vi "Ball Ball Velocity after Collision Calcul.vi"(10 "Movables in":refnum<class "Movable.lvclass">[](array[class])) -> (2 "Movables out":refnum<class "Movable.lvclass">[](array[class]))   [LabVIEW 2024, in "Game Board.lvclass"]
doc: "MIT Licence\nCopyright (c) 2024 David Grollier"
uses:
  Game Board.lvclass
  Game Board Component/Movable/Movable.lvclass
  Game Board Component/Movable/Movable.lvclass/Movable.ctl
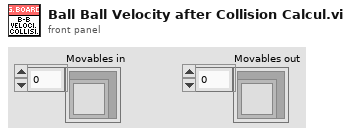
[diagram p1: front panel]
types:
  T1 = typedef "Coordinates.ctl" = cluster{"x":dbl, "y":dbl}
  T2 = typedef "Velocity.ctl" = cluster{"Vx":dbl, "Vy":dbl}
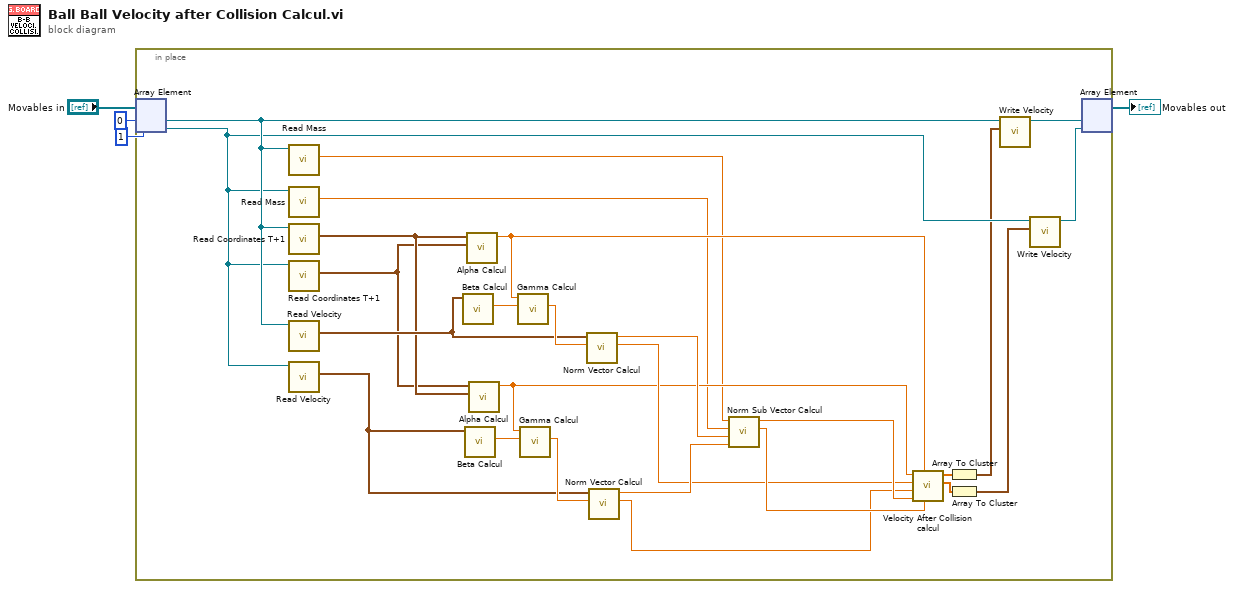
[diagram p0: block diagram]
diagram:
  n1 = in-place {
    n2 = in-place-array #1("Movables in", 0, 1) -> (w12:refnum<class "Movable.lvclass">, w11:refnum<class "Movable.lvclass">)
    n3 = call "Read Mass.vi"("Movable in"=w12) -> ("Mass"=w16:dbl)  [unwired: 10 in]
    n4 = call "Read Mass.vi"("Movable in"=w11) -> ("Mass"=w15:dbl)  [unwired: 10 in]
    n5 = call "Read Coordinates T+1.vi"("Movable in"=w12) -> ("Coordinates"=w9:T1)  [unwired: 10 in]
    n6 = call "Read Coordinates T+1.vi"("Movable in"=w11) -> ("Coordinates"=w7:T1)  [unwired: 10 in]
    n7 = call-dynamic "Read Velocity.vi"("Movable in"=w12) -> ("Velocity"=w14:T2)  [unwired: 10 in]
    n8 = call-dynamic "Read Velocity.vi"("Movable in"=w11) -> ("Velocity"=w13:T2)  [unwired: 10 in]
    n9 = call "Beta Calcul.vi"("Velocity in"=w14) -> ("Beta out"=w29:dbl)  [unwired: 10 in]
    n10 = call "Beta Calcul.vi"("Velocity in"=w13) -> ("Beta out"=w26:dbl)  [unwired: 10 in]
    n11 = call "Alpha Calcul.vi"("Coordinates 2 in"=w7, "Coordinates 1 in"=w9) -> ("Alpha out"=w20:dbl)  [unwired: 9 in]
    n12 = call "Alpha Calcul.vi"("Coordinates 2 in"=w9, "Coordinates 1 in"=w7) -> ("Alpha out"=w19:dbl)  [unwired: 9 in]
    n13 = call "Gamma Calcul.vi"("Beta in"=w29, "Alpha in"=w20) -> ("Gamma out"=w28:dbl)  [unwired: 9 in]
    n14 = call "Gamma Calcul.vi"("Beta in"=w26, "Alpha in"=w19) -> ("Gamma out"=w27:dbl)  [unwired: 9 in]
    n15 = call "Norm Vector Calcul.vi"("Gamma"=w28, "Velocity in"=w14) -> ("Vector u11/22"=w21:dbl, "Vector u21/12"=w24:dbl)  [unwired: 8 in]
    n16 = call "Norm Vector Calcul.vi"("Gamma"=w27, "Velocity in"=w13) -> ("Vector u11/22"=w22:dbl, "Vector u21/12"=w25:dbl)  [unwired: 8 in]
    n17 = call "Norm Sub Vector Calcul.vi"("u21"=w25, "u12"=w24, "m2"=w15, "m1"=w16) -> ("v21"=w30:dbl, "v12"=w23:dbl)  [unwired: 6 in]
    n18 = call "Velocity After Collision calcul.vi"("v21"=w30, "Alpha1 in"=w20, "v12"=w23, "u22"=w22, "u11"=w21, "Alpha2 in"=w19) -> ("V2 out"=w17:dbl[], "V1 out"=w18:dbl[])  [unwired: 4 in]
    n19 = Array To Cluster(array=w18) -> (cluster=w10:cluster{"V1 out[0]":dbl, "V1 out[1]":dbl})
    n20 = Array To Cluster(array=w17) -> (cluster=w8:cluster{"V2 out[0]":dbl, "V2 out[1]":dbl})
    n21 = call "Write Velocity.vi"("Velocity"=w10, "Movable in"=w12) -> ("Movable out"=w5:refnum<class "Movable.lvclass">)  [unwired: 9 in]
    n22 = call "Write Velocity.vi"("Velocity"=w8, "Movable in"=w11) -> ("Movable out"=w6:refnum<class "Movable.lvclass">)  [unwired: 9 in]
    n23 = in-place-array #1(w5, w6) -> (→"Movables out":refnum<class "Movable.lvclass">[])  [unwired: 2 out]
  }
